vi "CarWashControllerServer.vi"() -> ()   [LabVIEW 2021]
uses:
  <vilib>/Utility/file.llb/Read Delimited Spreadsheet (string).vi
  <vilib>/Utility/file.llb/Write Delimited Spreadsheet (string).vi
panel:
  in  "file path (dialog if empty)":path
  out "tblCarWash":string[][](table)
  out "LED-washInProgressEntrance(F)":bool
  out "LED-washInProgressEntrance(T)":bool
  out "LED-washInProgressExit(T)":bool
  out "LED-washInProgressExit(F)":bool
  out "LED-MWCycle":bool
  out "LED-AD Cycle":bool
  out "LED-UWCycle":bool
  out "error out":errorcluster
  # "Car Wash Details"
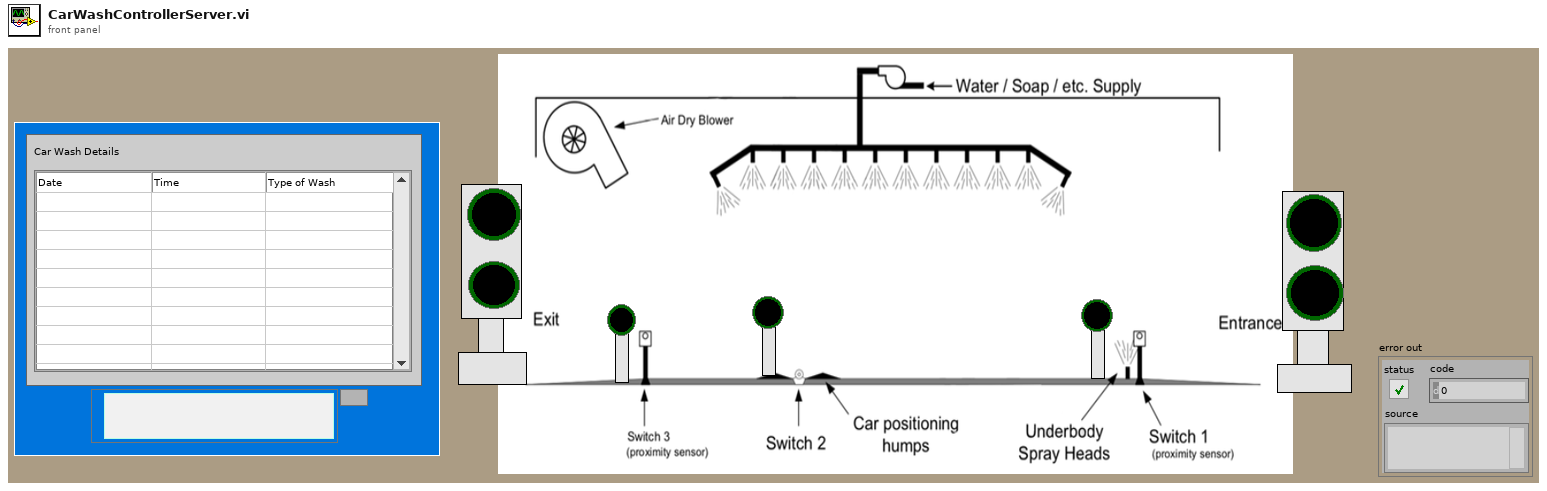
[diagram p1: front panel]
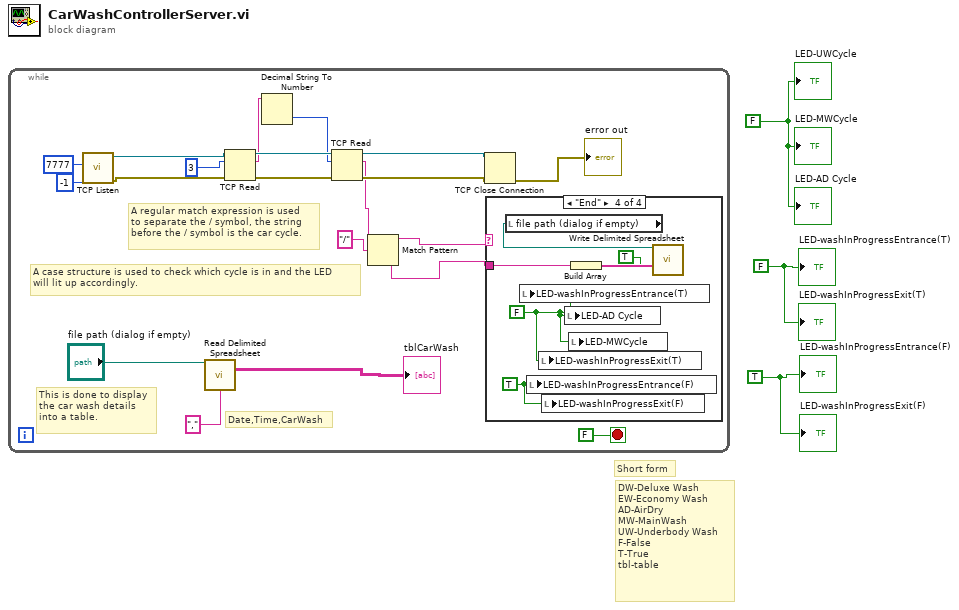
[diagram p0: block diagram]
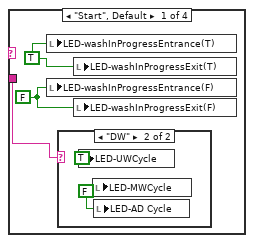
[diagram p2: hidden frame]
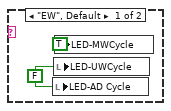
[diagram p3: hidden frame]
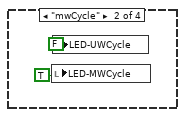
[diagram p4: hidden frame]
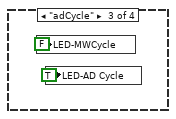
[diagram p5: hidden frame]
diagram:
  w2 = TRUE ("LED-washInProgressEntrance(F)")
  w1 = FALSE ("LED-washInProgress")
  w3 = FALSE ("cycle1")
  # "Short form"
  # "DW-Deluxe Wash\nEW-Economy Wash\nAD-AirDry\nMW-MainWash\nUW-Underbody Wash\nF-False\nT-True\ntbl-table"
  n1 = while {
    stop <- FALSE stop-if-true
    # "This is done to display\nthe car wash details\ninto a table."
    # "A case structure is used to check which cycle is in and the LED\nwill lit up accordingly."
    # "A regular match expression is used\nto separate the / symbol, the string\nbefore the / symbol is the car cycle."
    # "Date,Time,CarWash"
    n2 = call <vilib>:"TCP Listen.vi"("timeout ms (wait forever: -1)"=-1, "port"=u16 7777) -> ("error out"=w20:errorcluster, "connection ID"=w21:refnum<k5>)  [unwired: 5 in, 3 out]
    n3 = call-poly <vilib>:"Read Delimited Spreadsheet.vi"("file path (dialog if empty)"="file path (dialog if empty)", "delimiter (\\t)"="," ("delimiter (\\t)")) -> ("all rows"=→"tblCarWash":string[][])  [unwired: 8 in, 5 out]
    n4 = TCP Read(connection ID=w21, bytes to read=3 ("timeout ms (25000)"), error in (no error)=w20) -> (connection ID out=w18:refnum<k5>, data out=w14:string, error out=w17:errorcluster)  [unwired: 2 in]
    n5 = Decimal String To Number(string=w14) -> (number=w13:i32)  [unwired: 2 in, 1 out]
    n6 = TCP Read(connection ID=w18, bytes to read=w13, error in (no error)=w17) -> (connection ID out=w16:refnum<k5>, data out=w7:string, error out=w15:errorcluster)  [unwired: 2 in]
    n7 = Match Pattern(string=w7, regular expression="/") -> (before substring=w5:string, after substring=w4:string)  [unwired: 1 in, 2 out]
    n8 = TCP Close Connection(connection ID=w16, error in (no error)=w15) -> (error out=→"error out":errorcluster)  [unwired: 1 in, 1 out]
    n9 = case shown="\"End\"" w5 {
      tunnel: w4 -> [w26 _ _ w37]
      frame "Start", Default {
        w24 = FALSE ("LED-washInProgressEntrance(F)")
        w25 = TRUE ("LED-washInProgress")
        n10 = local write "LED-washInProgressEntrance(T)"(w25) -> ()
        n11 = local write "LED-washInProgressEntrance(F)"(w24) -> ()
        n12 = case shown="\"DW\"" w26 {
          frame "EW", Default {
            w27 = FALSE ("cycle1")
            n13 = local write "LED-AD Cycle"(w27) -> ()
            n14 = local write "LED-UWCycle"(w27) -> ()
            n15 = local write "LED-MWCycle"(TRUE ("cycle2")) -> ()
          }
          frame "DW" {
            w29 = FALSE ("cycle2")
            n16 = local write "LED-UWCycle"(TRUE ("cycle1")) -> ()
            n17 = local write "LED-MWCycle"(w29) -> ()
            n18 = local write "LED-AD Cycle"(w29) -> ()
          }
        }
        n19 = local write "LED-washInProgressExit(T)"(w25) -> ()
        n20 = local write "LED-washInProgressExit(F)"(w24) -> ()
      }
      frame "mwCycle" {
        n21 = local write "LED-MWCycle"(TRUE ("cycle2")) -> ()
        n22 = local write "LED-UWCycle"(FALSE ("cycle1")) -> ()
      }
      frame "adCycle" {
        n23 = local write "LED-MWCycle"(FALSE ("cycle2")) -> ()
        n24 = local write "LED-AD Cycle"(TRUE ("cycle3")) -> ()
      }
      frame "End" {
        w35 = TRUE ("LED-washInProgressEntrance(F)")
        w36 = FALSE ("LED-washInProgress")
        n25 = local read "file path (dialog if empty)"() -> (w39:path)
        n26 = local write "LED-washInProgressEntrance(T)"(w36) -> ()
        n27 = local write "LED-washInProgressEntrance(F)"(w35) -> ()
        n28 = local write "LED-washInProgressExit(T)"(w36) -> ()
        n29 = local write "LED-washInProgressExit(F)"(w35) -> ()
        n30 = local write "LED-AD Cycle"(w36) -> ()
        n31 = local write "LED-MWCycle"(w36) -> ()
        n32 = Build Array "Build Array"(w37) -> (w40:string[])
        n33 = call-poly <vilib>:"Write Delimited Spreadsheet.vi"("file path (dialog if empty)"=w39, "1D data"=w40, "append to file? (new file:F)"=TRUE) -> ()  [unwired: 11 in, 2 out]
      }
    }
  }
  "LED-washInProgressEntrance(T)" <- w1
  "LED-AD Cycle" <- w3
  "LED-MWCycle" <- w3
  "LED-UWCycle" <- w3
  "LED-washInProgressExit(F)" <- w2
  "LED-washInProgressExit(T)" <- w1
  "LED-washInProgressEntrance(F)" <- w2
